vi "Save.vi"(8 "error in (no error)":errorcluster, 10 "Model Path":path, 11 "MarkovModel in":refnum<class "MarkovModel.lvclass">) -> (0 "error out":errorcluster, 3 "MarkovModel out":refnum<class "MarkovModel.lvclass">)   [LabVIEW 2024, in "MarkovModel.lvclass"]
uses:
  MarkovModel.lvclass
  MarkovModel.lvclass/MarkovModel.ctl
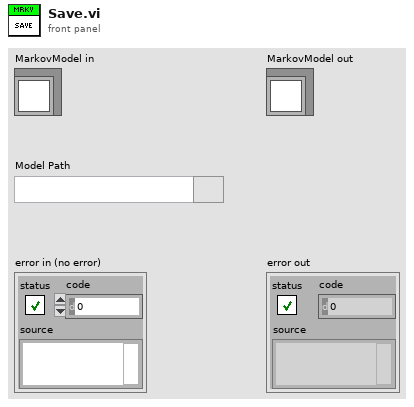
[diagram p1: front panel]
types:
  T1 = map{string[], cluster{"Class Name":string, "Count":i32}[]}
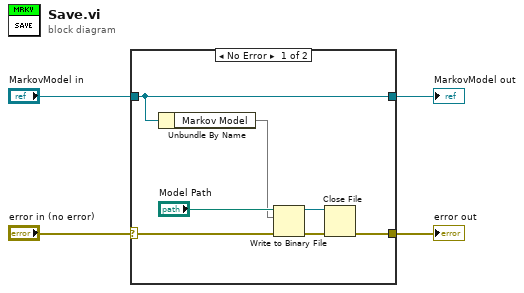
[diagram p0: block diagram]
diagram:
  n1 = case shown="No Error" "error in (no error)" {
    selector: "error in (no error)" -> [w9 w13]
    tunnel: [w8 w13] -> w3
    tunnel: "MarkovModel in" -> [w7 w12]
    tunnel: [w7 w12] -> w1
    frame No Error {
      n2 = Unbundle By Name(w7) -> ("Markov Model"=w5:T1)
      n3 = Write to Binary File(file (use dialog)="Model Path", data=w5, error in=w9) -> (refnum out=w10:refnum<file>, error out=w11:errorcluster)  [unwired: 3 in, 1 out]
      n4 = Close File(refnum=w10, error in=w11) -> (error out=w8:errorcluster)  [unwired: 1 out]
    }
    frame Error {
    }
  }
  "error out" <- w3
  "MarkovModel out" <- w1
